vi "AT Unregister Feature Callback A.vi"(8 "error in (no error)":errorcluster, 9 "Event":refnum<user-event>, 10 "Feature":string, 11 "Handle":i32) -> (0 "error out":errorcluster, 3 "Status":i32)   [LabVIEW 2009]
doc: "Unregister Feature Callback\n\nOutput:\n I32 Status\n\nInput:\n I32 Handle\n String Feature\n UserEvent Event\n\nDescription\nThis function is used to un-register a callback event previously registered using AT_RegisterFeatureCallback. The same parameters that were passed to the register function should be passed to this unregister function. Once this function is called, no more callbacks will be sent to this callback function for the specified Feature."
uses:
  atlvcallbacks.dll
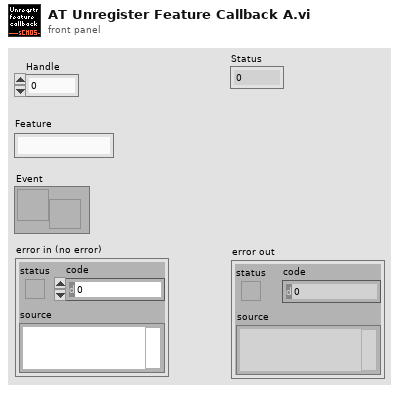
[diagram p1: front panel]
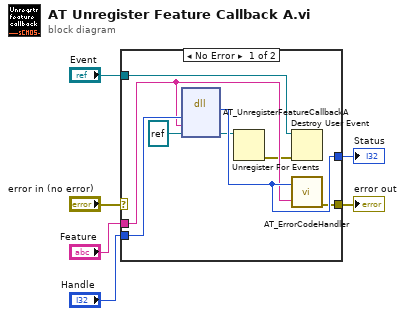
[diagram p0: block diagram]
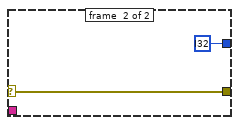
[diagram p2: hidden frame]
diagram:
  n1 = case shown="No Error" "error in (no error)" {
    selector: "error in (no error)" -> [_ w16]
    tunnel: "Feature" -> [w12 _]
    tunnel: "Handle" -> [w14 _]
    tunnel: [w13 i32 ? ("Status")] -> w3
    tunnel: [w11 w16] -> w2
    tunnel: "Event" -> [w7 _]
    frame #0 {
      n2 = dll-call lib="atlvcallbacks.dll" fn="AT_UnregisterFeatureCallbackA"("Handle"=w14, "Feature"=w12, "Event"=refnum<event-registration> ? ("event registration refnum")) -> ("Status"=w13:i32, "Event"=w9:refnum<event-registration>)  [unwired: 5 in, 2 out]
      n3 = Unregister For Events(event registration refnum=w9) -> (error out=w8:errorcluster)  [unwired: 1 in]
      n4 = Destroy User Event(user event=w7, error in=w8) -> ()  [unwired: 1 out]
      n5 = call "AT_ErrorCodeHandler.vi"("Error"=w13, "Feature Name"=w12) -> ("error out"=w11:errorcluster)  [unwired: 5 in]
    }
    frame #1 {
    }
  }
  "error out" <- w2
  "Status" <- w3
